vi "Wave1D_Init Data_Start Idx and Length.vi"(10 "Boundary Condition":cluster{"type":T2, "Value":dbl[]}[](array[cluster]) {"type" items=["Dirichlet", "Neumann"]}, 11 "Domain":T1={"t"={"initial t"=0.0, "final t"=1.0, "# of t-points"=11}, "x"={"start x"=0.0, "end x"=1.0, "# of x-points"=11}}) -> (2 "length":i32, 3 "start index":i32)   [LabVIEW 2020, in "NI_PDE.lvlib"]
uses:
  <vilib>/gmath/NI_PDE.lvlib
  <vilib>/gmath/pde.llb/Common/PDE_BC Type.ctl
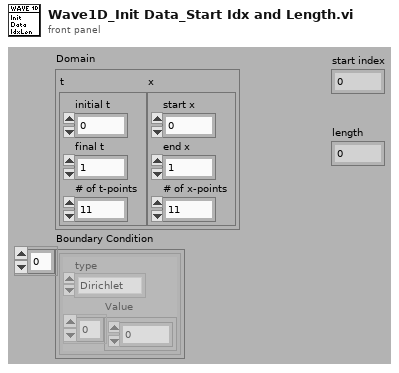
[diagram p1: front panel]
types:
  T1 = cluster{"t":cluster{"initial t":dbl, "final t":dbl, "# of t-points":i32}, "x":cluster{"start x":dbl, "end x":dbl, "# of x-points":i32}}
  T2 = typedef "NI_PDE.lvlib/PDE_BC Type.ctl" = i32
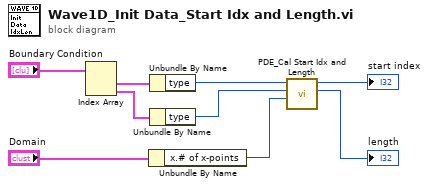
[diagram p0: block diagram]
diagram:
  n1 = Index Array(array="Boundary Condition") -> (element #1=w8:cluster{"type":T2, "Value":dbl[]}, element #2=w7:cluster{"type":T2, "Value":dbl[]})  [unwired: 2 in]
  n2 = Unbundle By Name("Domain") -> ("x.# of x-points"=w3:i32)
  n3 = Unbundle By Name(w8) -> ("type"=w5:T2)
  n4 = Unbundle By Name(w7) -> ("type"=w4:T2)
  n5 = call <vilib>:"PDE_Cal Start Idx and Length.vi"("# of points"=w3, "end type"=w4, "start type"=w5) -> ("length"=→"length":i32, "start index"=→"start index":i32)  [unwired: 7 out]
